vi "PORT IO VI Tree__ogtk.vi"   [LabVIEW 2012]
panel:
  # "[OpenG VI Tags] ***Do Not Remove***"
  # "PORT IO VI Tree.vi\n\nPlease visit http://www.OpenG.org to learn about the\nOpen Source LabVIEW software movement.\n\nNOTICE -- YOU MUST LEAVE THIS NOTICE IN PLACE.  PER THE TERMS OF THE LICENSE BELOW, YOU MAY SUBLICENSE THIS SOFTWARE \nIN ANY WAY THAT DOES NOT CONFLICT WITH THIS LICENSE.\n\n### BSD License (http://www.opensource.org/licenses/bsd-license.php) Begin ###\n\nCopyright (c) 2002-2007, Rolf Kalbermatter <rolf.kalbermatter@citeng.com> \n\nAll rights reserved.\n\nRedistribution and use in source and binary forms, with or without modification, are permitted provided that the following conditions are met:\n\n    * Redistributions of source code must retain the above copyright notice, this list of conditions and the following disclaimer.\n    * Redistributions in binary form must reproduce the above copyright notice, this list of conditions and the following disclaimer in the \n       documentation and/or other materials provided with the distribution.\n    * Neither the name of SciWare, James Kring, Inc., nor the names of its contributors may be used to endorse or promote products derived \n       from this software without specific prior written permission.\n\nTHIS SOFTWARE IS PROVIDED BY THE COPYRIGHT HOLDERS AND CONTRIBUTORS \"AS IS\" AND ANY EXPRESS OR IMPLIED WARRANTIES, \nINCLUDING, BUT NOT LIMITED TO, THE IMPLIED WARRANTIES OF MERCHANTABILITY AND FITNESS FOR A PARTICULAR PURPOSE ARE \nDISCLAIMED. IN NO EVENT SHALL THE COPYRIGHT OWNER OR CONTRIBUTORS BE LIABLE FOR ANY DIRECT, INDIRECT, INCIDENTAL,\n SPECIAL, EXEMPLARY, OR CONSEQUENTIAL DAMAGES (INCLUDING, BUT NOT LIMITED TO, PROCUREMENT OF SUBSTITUTE GOODS OR \nSERVICES; LOSS OF USE, DATA, OR PROFITS; OR BUSINESS INTERRUPTION) HOWEVER CAUSED AND ON ANY THEORY OF LIABILITY, \nWHETHER IN CONTRACT, STRICT LIABILITY, OR TORT (INCLUDING NEGLIGENCE OR OTHERWISE) ARISING IN ANY WAY OUT OF THE USE \nOF THIS SOFTWARE, EVEN IF ADVISED OF THE POSSIBILITY OF SUCH DAMAGE.\n\n### BSD License End ###"
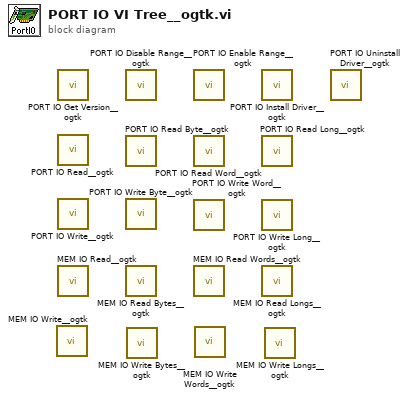
[diagram p0: block diagram]
diagram:
  n1 = call-poly <userlib>:"MEM IO Write__ogtk.vi"() -> ()  [unwired: 7 in, 1 out]
  n2 = call <userlib>:"PORT IO Get Version__ogtk.vi"() -> ()  [unwired: 6 in, 2 out]
  n3 = call-poly <userlib>:"PORT IO Read__ogtk.vi"() -> ()  [unwired: 6 in, 2 out]
  n4 = call-poly <userlib>:"PORT IO Write__ogtk.vi"() -> ()  [unwired: 7 in, 1 out]
  n5 = call-poly <userlib>:"MEM IO Read__ogtk.vi"() -> ()  [unwired: 6 in, 2 out]
  n6 = call <userlib>:"PORT IO Disable Range__ogtk.vi"() -> ()  [unwired: 7 in, 1 out]
  n7 = call <userlib>:"PORT IO Read Byte__ogtk.vi"() -> ()  [unwired: 6 in, 2 out]
  n8 = call <userlib>:"PORT IO Write Byte__ogtk.vi"() -> ()  [unwired: 7 in, 1 out]
  n9 = call <userlib>:"MEM IO Read Bytes__ogtk.vi"() -> ()  [unwired: 6 in, 2 out]
  n10 = call <userlib>:"MEM IO Write Bytes__ogtk.vi"() -> ()  [unwired: 7 in, 1 out]
  n11 = call <userlib>:"PORT IO Enable Range__ogtk.vi"() -> ()  [unwired: 7 in, 1 out]
  n12 = call <userlib>:"PORT IO Read Word__ogtk.vi"() -> ()  [unwired: 6 in, 2 out]
  n13 = call <userlib>:"PORT IO Write Word__ogtk.vi"() -> ()  [unwired: 7 in, 1 out]
  n14 = call <userlib>:"MEM IO Read Words__ogtk.vi"() -> ()  [unwired: 6 in, 2 out]
  n15 = call <userlib>:"MEM IO Write Words__ogtk.vi"() -> ()  [unwired: 7 in, 1 out]
  n16 = call <userlib>:"PORT IO Install Driver__ogtk.vi"() -> ()  [unwired: 7 in, 1 out]
  n17 = call <userlib>:"PORT IO Read Long__ogtk.vi"() -> ()  [unwired: 6 in, 2 out]
  n18 = call <userlib>:"PORT IO Write Long__ogtk.vi"() -> ()  [unwired: 7 in, 1 out]
  n19 = call <userlib>:"MEM IO Read Longs__ogtk.vi"() -> ()  [unwired: 6 in, 2 out]
  n20 = call <userlib>:"MEM IO Write Longs__ogtk.vi"() -> ()  [unwired: 7 in, 1 out]
  n21 = call <userlib>:"PORT IO Uninstall Driver__ogtk.vi"() -> ()  [unwired: 7 in, 1 out]
